vi "Interpolate Trajectory States.vi"(9 "timestamp":dbl, 10 "State [n]":T1, 11 "State [n-1]":T1) -> (3 "Interpolated State":T1)   [LabVIEW 2019]
uses:
  Typedef/Trajectory State.ctl
  Geometry/Typedef/Pose2d.ctl
  Geometry/Typedef/Translation2d.ctl
  Geometry/Typedef/Rotation2d.ctl
  81649ad7-b5e7-4926-a093-485b6a7d21e2.vi
  a3143a93-a4c7-4e51-b6db-09cae8a3661f.vi
  81649ad7-b5e7-4926-a093-485b6a7d21e2.vi/daf58034-9565-4719-9f2c-6764e5c93ab4.vi
  a3143a93-a4c7-4e51-b6db-09cae8a3661f.vi/2858566f-cb51-4dea-b8b8-9ca3c535ce89.vi
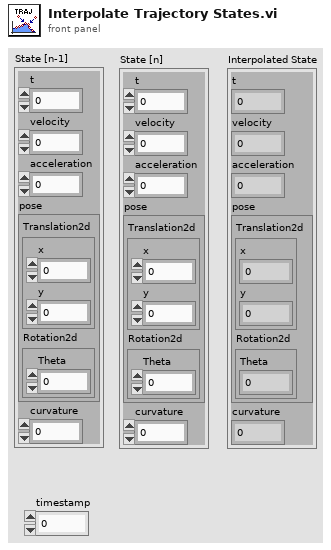
[diagram p1: front panel]
types:
  T1 = typedef "Trajectory State.ctl" = cluster{"t":dbl, "velocity":dbl, "acceleration":dbl, "pose":T2, "curvature":dbl}
  T2 = typedef "Pose2d.ctl" = cluster{"Translation2d":T3, "Rotation2d":T4}
  T3 = typedef "Translation2d.ctl" = cluster{"x":dbl, "y":dbl}
  T4 = typedef "Rotation2d.ctl" = cluster{"Theta":dbl}
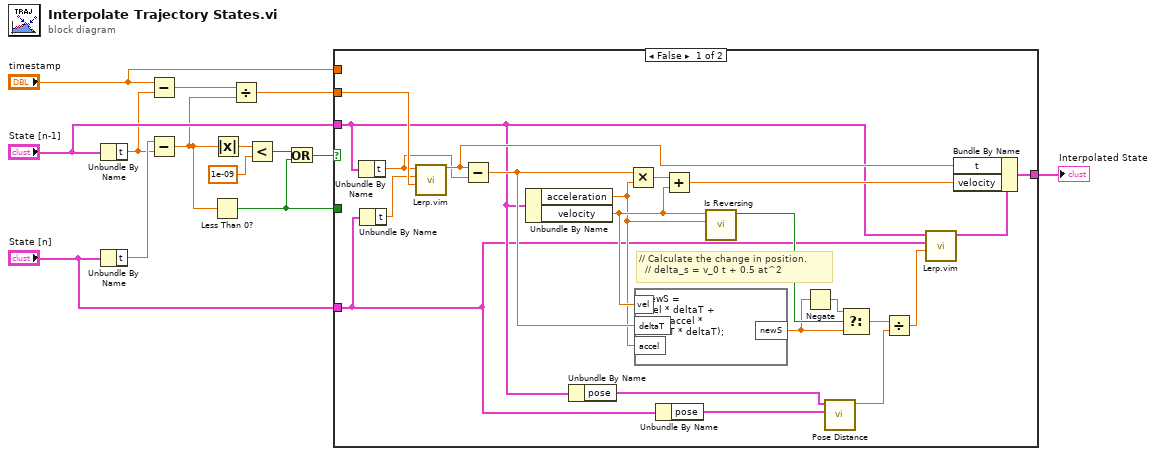
[diagram p0: block diagram]
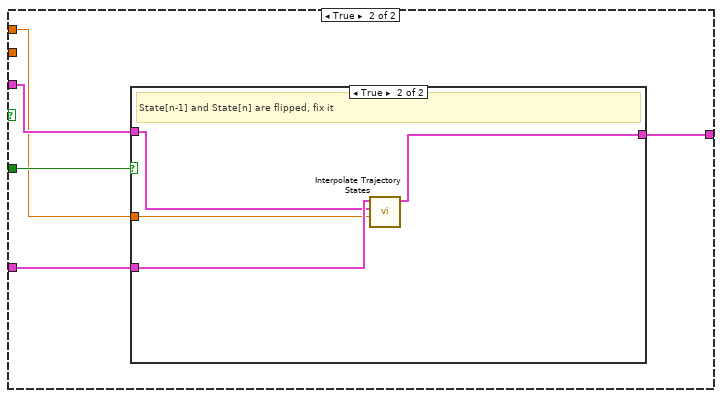
[diagram p2: hidden frame]
diagram:
  n1 = Unbundle By Name("State [n-1]") -> ("t"=w7:dbl)
  n2 = Unbundle By Name("State [n]") -> ("t"=w14:dbl)
  n3 = Subtract(x="timestamp", y=w7) -> (x-y=w6:dbl)
  n4 = Subtract(x=w14, y=w7) -> (x-y=w3:dbl)
  n5 = Less Than 0?(x=w3) -> (x < 0?=w2:bool)
  n6 = Absolute Value(x=w3) -> (abs(x)=w13:dbl)
  n7 = Divide(x=w6, y=w3) -> (x/y=w5:dbl)
  n8 = Less?(x=w13, y=1e-09) -> (x < y?=w11:bool)
  n9 = Or(x=w11, y=w2) -> (x .or. y?=w4:bool)
  n10 = case shown="False" w4 {
    tunnel: "State [n]" -> [w15 w40]
    tunnel: [w35 w38] -> w9
    tunnel: "State [n-1]" -> [w16 w37]
    tunnel: w5 -> [w32 _]
    tunnel: w2 -> [_ w39]
    tunnel: "timestamp" -> [_ w36]
    frame False {
      # "// Calculate the change in position.\n  // delta_s = v_0 t + 0.5 at^2"
      n11 = Unbundle By Name(w16) -> ("t"=w19:dbl)
      n12 = Unbundle By Name(w15) -> ("t"=w20:dbl)
      n13 = call "Lerp.vim"("Percent"=w32, "Y"=w20, "X"=w19) -> ("Output"=w33:dbl)  [unwired: 8 in]
      n14 = Subtract(x=w33, y=w19) -> (x-y=w34:dbl)
      n15 = Unbundle By Name(w16) -> ("acceleration"=w25:dbl, "velocity"=w26:dbl)
      n16 = Unbundle By Name(w16) -> ("pose"=w18:T2)
      n17 = Multiply(x=w34, y=w25) -> (x*y=w31:dbl)
      n18 = formula code="newS = \n(vel * deltaT + \n0.5 * accel * \ndeltaT * deltaT);"("vel"=w26, "deltaT"=w34, "accel"=w25) -> ("newS"=w27:dbl)
      n19 = Unbundle By Name(w15) -> ("pose"=w17:T2)
      n20 = Add(x=w31, y=w26) -> (x+y=w30:dbl)
      n21 = call "Is Reversing.vi"("acceleration"=w25, "velocity"=w26) -> ("Reversing?"=w29:bool)  [unwired: 9 in]
      n22 = Negate(x=w27) -> (-x=w28:dbl)
      n23 = call "Pose Distance.vi"("Start Pose"=w17, "End Pose"=w18) -> ("Distance"=w21:dbl)  [unwired: 9 in]
      n24 = Select(t=w28, s=w29, f=w27) -> (s? t:f=w24:dbl)
      n25 = Divide(x=w24, y=w21) -> (x/y=w22:dbl)
      n26 = call "Lerp.vim"("Percent"=w22, "Y"=w15, "X"=w16) -> ("Output"=w23:T1)  [unwired: 8 in]
      n27 = Bundle By Name(cluster=w23, "t"=w33, "velocity"=w30) -> (w35:T1)
    }
    frame True {
      n28 = case shown="True" w39 {
        tunnel: w40 -> [w41 w45]
        tunnel: [w41 w42] -> w38
        tunnel: w37 -> [_ w44]
        tunnel: w36 -> [_ w43]
        frame False {
          # "Close enough between to just pick one"
        }
        frame True {
          # "State[n-1] and State[n] are flipped, fix it"
          n29 = call "Interpolate Trajectory States.vi"("timestamp"=w43, "State [n]"=w44, "State [n-1]"=w45) -> ("Interpolated State"=w42:T1)  [unwired: 8 in]
        }
      }
    }
  }
  "Interpolated State" <- w9
